vi "HP34970A Conf Voltage.vi"(0 "VISA session":refnum<visa-resource-name>, 1 "Set/Check (F:Set)":bool, 2 "Check Parameter(1:Ap Min)":T3(ring)=enum."Aperture Min", 5 "DC/AC (F:DC)":bool, 7 "Autorange (F:OFF)":bool, 9 "Voltage Range (6:Max)":T1(ring)=enum."Maximum", 11 "error in (no error)":errorcluster, 12 "Channel List(empty)":string, 13 "Advanced Config (F/1/4/1/3)":T2={"Aperture Value (.4)"=0.4, "Aperture (1:Minimum)"=enum."Minimum", "NPLC (1)"=enum."1", "Bandwidth (3 Hz)"=enum."3 Hz", "Input Impedance (F:Fixed)"=FALSE, "Integration Time (F:Aperture)"=FALSE} {"Aperture Value (.4)" min=0.4 max=4.0 format="%.2f"}) -> (4 "dup VISA session":refnum<visa-resource-name>, 8 "Configuration?":string, 15 "error out":errorcluster)   [LabVIEW 2020]
doc: "This VI configures the instrument for advanced voltage measurements."
panel:
  # "Check\nSet"
  # "ON\nOFF"
  # "AC\nDC"
  # "Auto\nFixed"
  # "NPLC\nAperture"
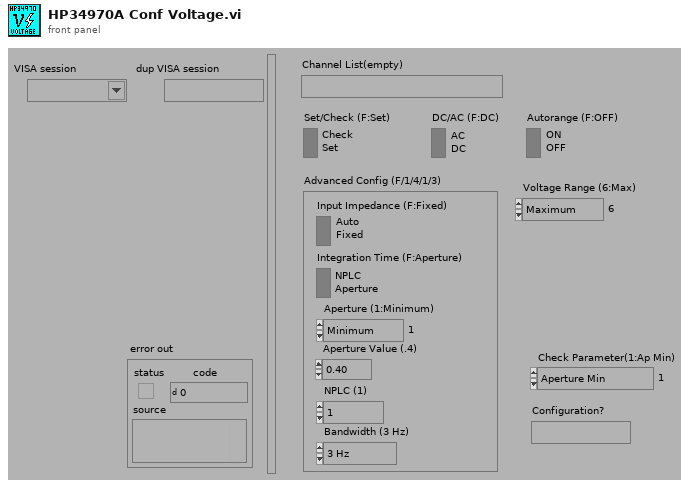
[diagram p1: front panel]
types:
  T1 = enum16{"100 mV", "1 V", "10 V", "100 V", "300 V", "Minimum", "Maximum"}
  T2 = cluster{"Aperture Value (.4)":dbl, "Aperture (1:Minimum)":enum16{"Manual", "Minimum", "Maximum"}, "NPLC (1)":enum16{".02", ".2", "1", "2", "10", "20", "100", "200", "Minimum", "Maximum"}, "Bandwidth (3 Hz)":enum16{"3 Hz", "20 Hz", "200 Hz", "Minimum", "Maximum"}, "Input Impedance (F:Fixed)":bool, "Integration Time (F:Aperture)":bool}
  T3 = enum16{"Aperture (By Chan)", "Aperture Min", "Aperture Max", "NPLC (By Chan)", "NPLC Min", "NPLC Max", "Bandwidth (By Chan)", "Bandwidth Min", "Bandwidth Max", "Impedance (By Chan)"}
  T4 = enum16{".02", ".2", "1", "2", "10", "20", "100", "200", "Minimum", "Maximum"}
  T5 = enum16{"3 Hz", "20 Hz", "200 Hz", "Minimum", "Maximum"}
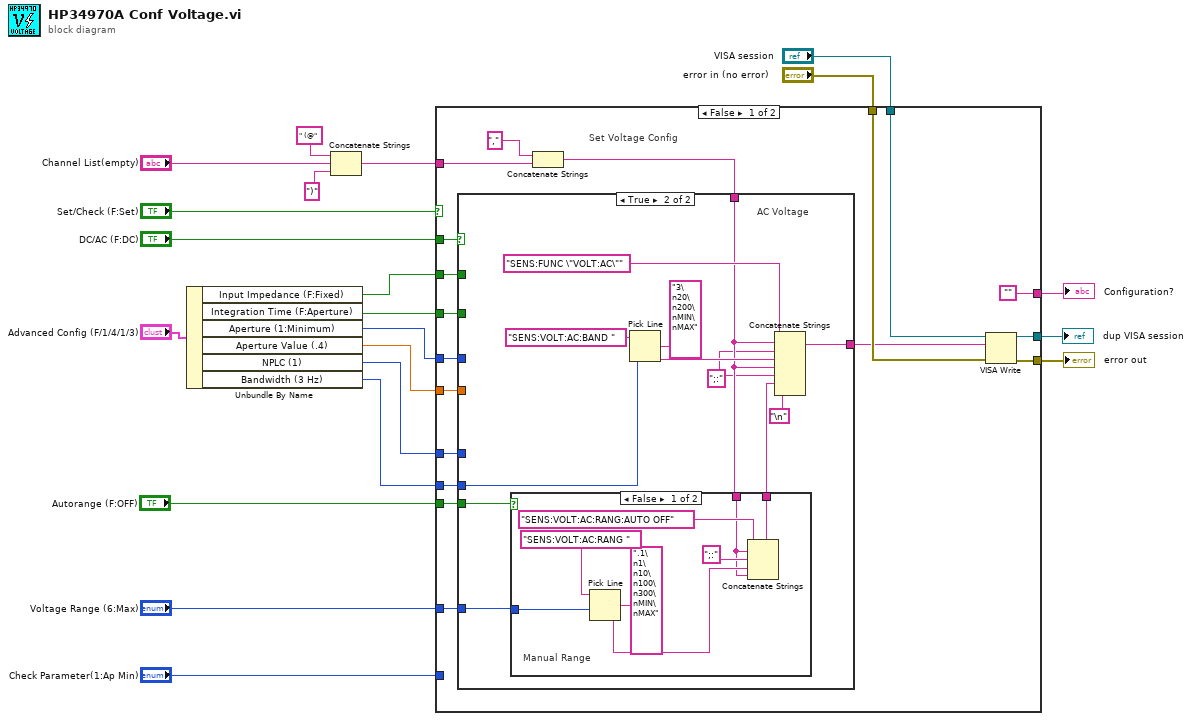
[diagram p0: block diagram]
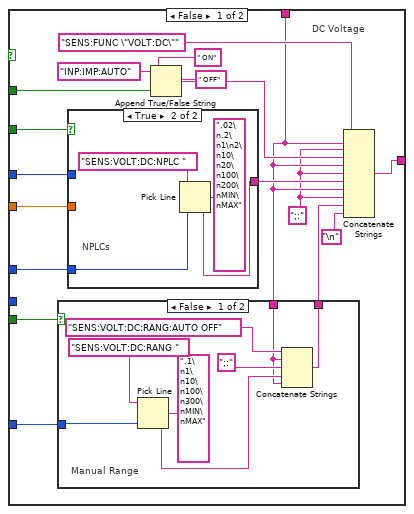
[diagram p2: hidden frame]
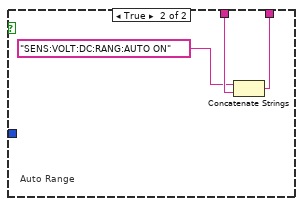
[diagram p3: hidden frame]
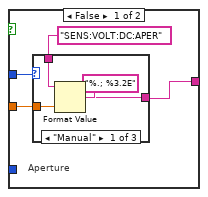
[diagram p4: hidden frame]
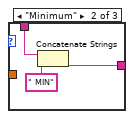
[diagram p5: hidden frame]
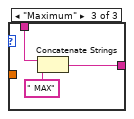
[diagram p6: hidden frame]
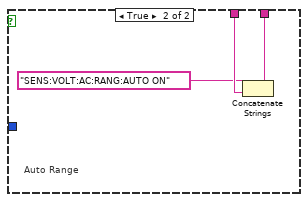
[diagram p7: hidden frame]
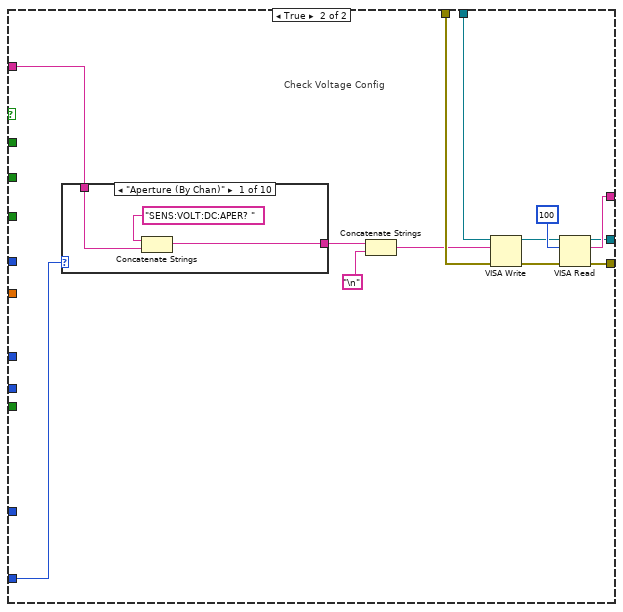
[diagram p8: hidden frame]
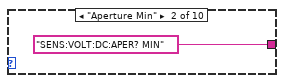
[diagram p9: hidden frame]
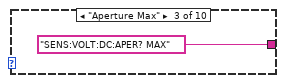
[diagram p10: hidden frame]
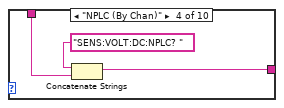
[diagram p11: hidden frame]
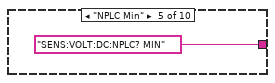
[diagram p12: hidden frame]
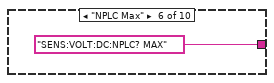
[diagram p13: hidden frame]
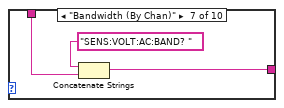
[diagram p14: hidden frame]
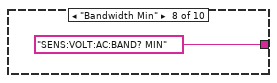
[diagram p15: hidden frame]
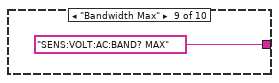
[diagram p16: hidden frame]
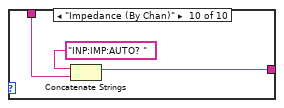
[diagram p17: hidden frame]
diagram:
  n1 = Unbundle By Name("Advanced Config (F/1/4/1/3)") -> ("Input Impedance (F:Fixed)"=w6:bool, "Integration Time (F:Aperture)"=w5:bool, "Aperture (1:Minimum)"=w4:enum16{"Manual", "Minimum", "Maximum"}, "Aperture Value (.4)"=w3:dbl, "NPLC (1)"=w2:T4, "Bandwidth (3 Hz)"=w1:T5)
  n2 = Concatenate Strings(" (@", "Channel List(empty)", ")") -> (w14:string)
  n3 = case shown="False" "Set/Check (F:Set)" {
    tunnel: [w26 w122] -> w20
    tunnel: [w27 w119] -> w21
    tunnel: "DC/AC (F:DC)" -> [w39 _]
    tunnel: w6 -> [w38 _]
    tunnel: w4 -> [w37 _]
    tunnel: w3 -> [w36 _]
    tunnel: w2 -> [w35 _]
    tunnel: w14 -> [w34 w113]
    tunnel: w1 -> [w31 _]
    tunnel: ["" w120] -> w13
    tunnel: "VISA session" -> [w29 w118]
    tunnel: "error in (no error)" -> [w28 w117]
    tunnel: "Check Parameter(1:Ap Min)" -> [_ w114]
    tunnel: w5 -> [w25 _]
    tunnel: "Autorange (F:OFF)" -> [w24 _]
    tunnel: "Voltage Range (6:Max)" -> [w23 _]
    frame False {
      # "Set Voltage Config"
      n4 = Concatenate Strings(",", w34) -> (w32:string)
      n5 = case shown="True" w39 {
        tunnel: w38 -> [w56 _]
        tunnel: w37 -> [w48 _]
        tunnel: w36 -> [w49 _]
        tunnel: w35 -> [w47 _]
        tunnel: w32 -> [w43 w90]
        tunnel: w31 -> [_ w95]
        tunnel: [w53 w94] -> w22
        tunnel: w25 -> [w50 _]
        tunnel: w24 -> [w45 w92]
        tunnel: w23 -> [w44 w91]
        frame False {
          w42 = ";:"
          # "DC Voltage"
          n6 = case shown="False" w45 {
            tunnel: w44 -> [w63 _]
            tunnel: w43 -> [w59 w68]
            tunnel: [w58 w66] -> w41
            frame False {
              # "Manual Range"
              n7 = Pick Line(string ("")="SENS:VOLT:DC:RANG ", multi-line string=".1\n1\n10\n100\n300\nMIN\nMAX", line index=w63) -> (output string=w60:string)
              n8 = Concatenate Strings("SENS:VOLT:DC:RANG:AUTO OFF", w59, ";:", w60, w59) -> (w58:string)
            }
            frame True {
              # "Auto Range"
              n9 = Concatenate Strings("SENS:VOLT:DC:RANG:AUTO ON", w68) -> (w66:string)
            }
          }
          n10 = case shown="True" w50 {
            tunnel: w49 -> [w71 _]
            tunnel: w48 -> [w70 _]
            tunnel: w47 -> [_ w84]
            tunnel: [w69 w83] -> w46
            frame False {
              # "Aperture"
              n11 = case shown="\"Manual\"" w70 {
                tunnel: "SENS:VOLT:DC:APER" -> [w76 w79 w81]
                tunnel: [w74 w77 w80] -> w69
                tunnel: w71 -> [w73 _ _]
                frame "Manual" {
                  n12 = Format Value(string ("")=w76, format string="%.; %3.2E", value (0)=w73) -> (output string=w74:string)
                }
                frame "Minimum" {
                  n13 = Concatenate Strings(w79, " MIN") -> (w77:string)
                }
                frame "Maximum" {
                  n14 = Concatenate Strings(w81, " MAX") -> (w80:string)
                }
              }
            }
            frame True {
              # "NPLCs"
              n15 = Pick Line(string ("")="SENS:VOLT:DC:NPLC ", multi-line string=".02\n.2\n1\n2\n10\n20\n100\n200\nMIN\nMAX", line index=w84) -> (output string=w83:string)
            }
          }
          n16 = Append True/False String(1:w56, 2:" OFF", 3:" ON", 4:"INP:IMP:AUTO") -> (0:w54:string)
          n17 = Concatenate Strings("SENS:FUNC \"VOLT:DC\"", w43, w42, w54, w43, w42, w46, w43, w42, w41, "\n") -> (w53:string)
        }
        frame True {
          w89 = ";:"
          # "AC Voltage"
          n18 = case shown="False" w92 {
            tunnel: w91 -> [w104 _]
            tunnel: w90 -> [w100 w109]
            tunnel: [w99 w107] -> w88
            frame False {
              # "Manual Range"
              n19 = Pick Line(string ("")="SENS:VOLT:AC:RANG ", multi-line string=".1\n1\n10\n100\n300\nMIN\nMAX", line index=w104) -> (output string=w101:string)
              n20 = Concatenate Strings("SENS:VOLT:AC:RANG:AUTO OFF", w100, ";:", w101, w100) -> (w99:string)
            }
            frame True {
              # "Auto Range"
              n21 = Concatenate Strings("SENS:VOLT:AC:RANG:AUTO ON", w109) -> (w107:string)
            }
          }
          n22 = Pick Line(string ("")="SENS:VOLT:AC:BAND ", multi-line string="3\n20\n200\nMIN\nMAX", line index=w95) -> (output string=w96:string)
          n23 = Concatenate Strings("SENS:FUNC \"VOLT:AC\"", w90, w89, w96, w90, w89, w88, "\n") -> (w94:string)
        }
      }
      n24 = VISA Write(VISA resource name=w29, write buffer=w22, error in (no error)=w28) -> (VISA resource name out=w27:refnum<visa-resource-name>, error out=w26:errorcluster)  [unwired: 1 out]
    }
    frame True {
      # "Check Voltage Config"
      n25 = case shown="\"Aperture (By Chan)\"" w114 {
        tunnel: w113 -> [w125 _ _ w129 _ _ w134 _ _ w139]
        tunnel: [w123 "SENS:VOLT:DC:APER? MIN" "SENS:VOLT:DC:APER? MAX" w128 "SENS:VOLT:DC:NPLC? MIN" "SENS:VOLT:DC:NPLC? MAX" w133 "SENS:VOLT:AC:BAND? MIN" "SENS:VOLT:AC:BAND? MAX" w138] -> w112
        frame "Aperture (By Chan)" {
          n26 = Concatenate Strings("SENS:VOLT:DC:APER? ", w125) -> (w123:string)
        }
        frame "Aperture Min" {
        }
        frame "Aperture Max" {
        }
        frame "NPLC (By Chan)" {
          n27 = Concatenate Strings("SENS:VOLT:DC:NPLC? ", w129) -> (w128:string)
        }
        frame "NPLC Min" {
        }
        frame "NPLC Max" {
        }
        frame "Bandwidth (By Chan)" {
          n28 = Concatenate Strings("SENS:VOLT:AC:BAND? ", w134) -> (w133:string)
        }
        frame "Bandwidth Min" {
        }
        frame "Bandwidth Max" {
        }
        frame "Impedance (By Chan)" {
          n29 = Concatenate Strings("INP:IMP:AUTO? ", w139) -> (w138:string)
        }
      }
      n30 = Concatenate Strings(w112, "\n") -> (w110:string)
      n31 = VISA Write(VISA resource name=w118, write buffer=w110, error in (no error)=w117) -> (VISA resource name out=w116:refnum<visa-resource-name>, error out=w115:errorcluster)  [unwired: 1 out]
      n32 = VISA Read(VISA resource name=w116, byte count=u32 100 ("byte count (0)"), error in (no error)=w115) -> (VISA resource name out=w119:refnum<visa-resource-name>, read buffer=w120:string, error out=w122:errorcluster)  [unwired: 1 out]
    }
  }
  "dup VISA session" <- w21
  "error out" <- w20
  "Configuration?" <- w13
